vi "q1 plot generation.vi"() -> ()   [LabVIEW 2018]
panel:
  in  "stop 2":bool
  out "Random Waveform Chart":cluster{dbl, dbl}(graph)
  in  "stop":bool
  out "random graph":dbl[](graph)
  out "random chart":dbl(graph)
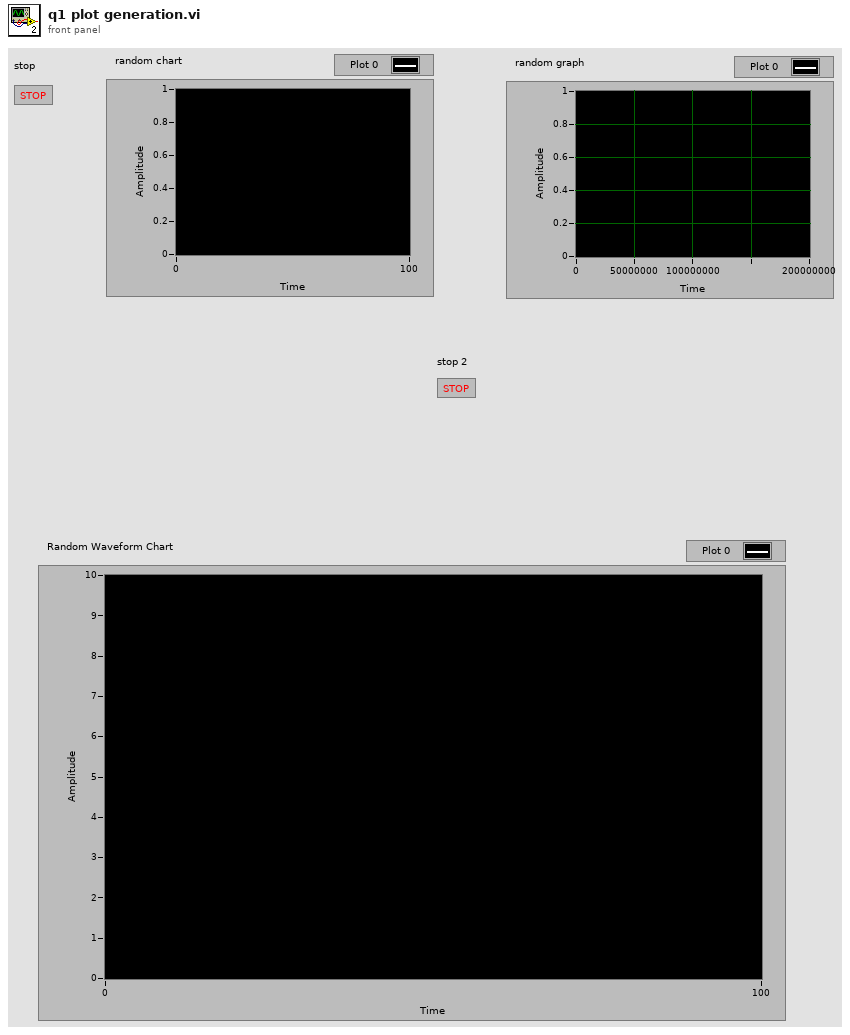
[diagram p1: front panel]
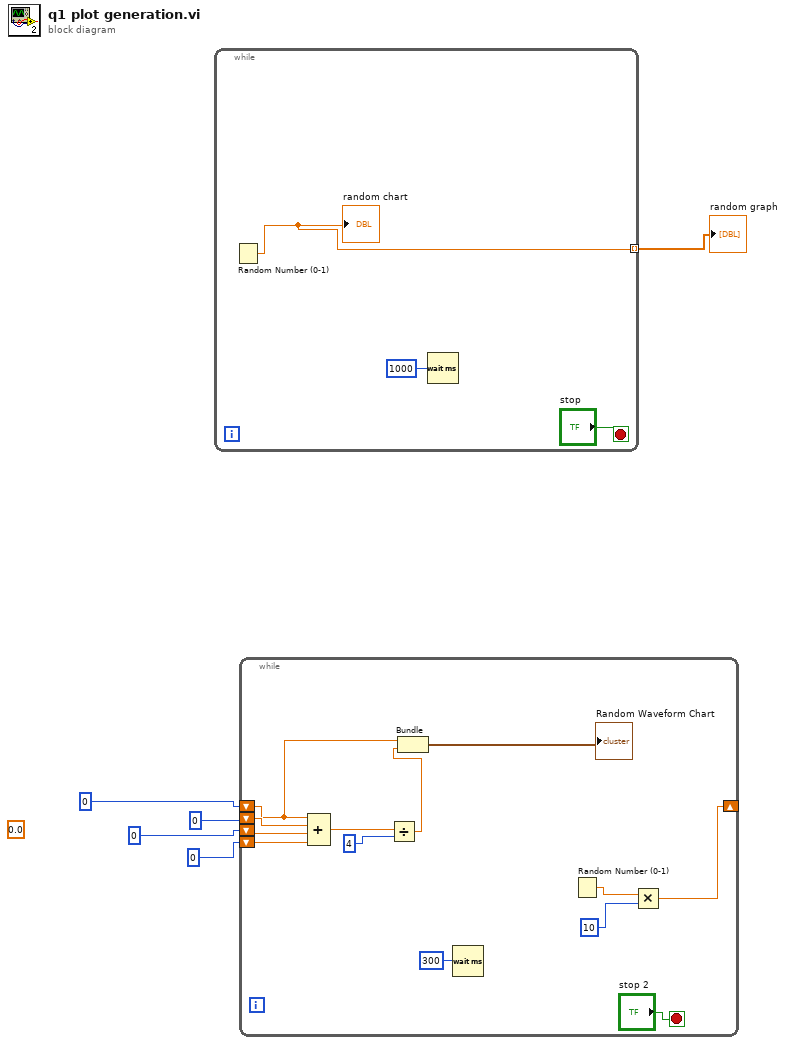
[diagram p0: block diagram]
diagram:
  (unwired) 0.0 ("Random Waveform Chart")
  n1 = while {
    tunnel: [w8] -> w5 mode=indexing
    stop <- "stop" stop-if-true
    n2 = Random Number (0-1)() -> (number: 0 to 1=w8:dbl)
    "random chart" <- w8
    n3 = Wait (ms)(milliseconds to wait=1000) -> ()  [unwired: 1 out]
  }
  "random graph" <- w5
  n4 = while {
    shift-right: [w10] -> _
    shift-left: 0 -> [w15]
    shift-left: 0 -> [w20]
    shift-left: 0 -> [w19]
    shift-left: 0 -> [w18]
    stop <- "stop 2" stop-if-true
    n5 = Compound Arithmetic op=ADD(w15, w20, w19, w18) -> (w17:dbl)
    n6 = Divide(x=w17, y=4) -> (x/y=w14:dbl)
    n7 = Bundle(w15, w14) -> (→"Random Waveform Chart":cluster{dbl, dbl})  [unwired: 1 in]
    n8 = Wait (ms)(milliseconds to wait=300) -> ()  [unwired: 1 out]
    n9 = Random Number (0-1)() -> (number: 0 to 1=w12:dbl)
    n10 = Multiply(x=w12, y=10) -> (x*y=w10:dbl)
  }
